vi "Render.vi"   [LabVIEW 2018, in "Toolkit.lvlib"]
doc: "Transverses an Abstract Syntax Tree (AST) obtained from the parsing process and writes the output based on the Mustache data. This is also known as \"code generation\" in compiling, and it is the third and final action, or process, in compiling."
uses:
  Toolkit.lvlib
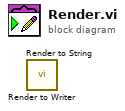
[diagram p0: block diagram]
diagram:
  n1 = call "Render to Writer.vi"() -> ()  [unwired: 10 in, 2 out]
  n2 = call "Render to String.vi"() -> ()  [unwired: 10 in, 2 out]
